vi "Filter Classes Descending from Test Case.vi"(8 "error in (no error)":errorcluster, 11 "Project Items":refnum<vi>[](array[refnum])) -> (0 "error out":errorcluster, 3 "Project Items out":refnum<vi>[](array[refnum]))   [LabVIEW 2020, in "Coverage Analyzer.lvclass"]
uses:
  Coverage Analyzer.lvclass
  Coverage Analyzer.lvclass/Coverage Analyzer.ctl
  Utilities/Utilities.lvlib
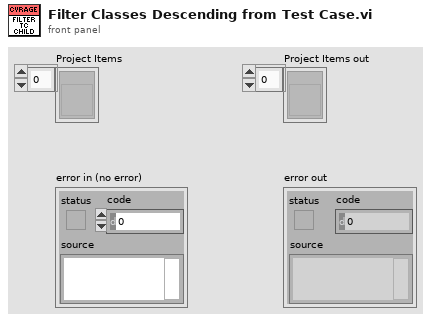
[diagram p1: front panel]
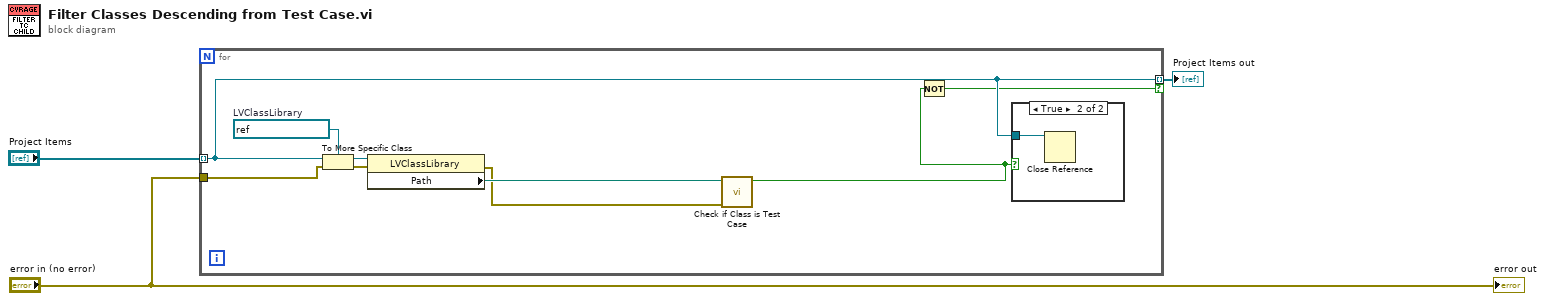
[diagram p0: block diagram]
diagram:
  n1 = for {
    tunnel: "Project Items" -> [w11] mode=indexing
    tunnel: "error in (no error)" -> [w12]
    tunnel: [w11] -> w1 mode=indexing if=w9
    w8 = refnum<vi> refnum  # LVClassLibrary
    n2 = To More Specific Class(target class=w8, reference=w11, error in=w12) -> (specific class reference=w7:refnum<vi>, error out=w4:errorcluster)
    n3 = property class="LVClassLibrary"(reference=w7, error in=w4) -> (error out=w5:errorcluster, "Path"=w6:path)  [unwired: 1 out]
    n4 = call "Check if Class is Test Case.vi"("error in (no error)"=w5, "Path"=w6) -> ("Is Test Case?"=w10:bool)  [unwired: 8 in, 1 out]
    n5 = Not(x=w10) -> (.not. x?=w9:bool)
    n6 = case shown="True" w10 {
      tunnel: w11 -> [_ w13]
      frame False {
      }
      frame True {
        n7 = Close Reference(reference=w13) -> ()  [unwired: 1 in, 1 out]
      }
    }
  }
  "Project Items out" <- w1
  "error out" <- "error in (no error)"
